vi "Close.vi"(8 "error in (no error)":errorcluster, 11 "MelsecTCP in":refnum<class "Abs Controler.lvclass">) -> (0 "error out":errorcluster, 3 "MelsecTCP out":refnum<class "Abs Controler.lvclass">)   [LabVIEW 2020, in "HslCommunication.lvlib" / "Abs Controler.lvclass"]
uses:
  Abs Controler.lvclass
  E:/Git/Libraries/develop/HslCommunication/_Dependenciecs/HslCommunication.dll
  _Dependenciecs/HslCommunication.dll
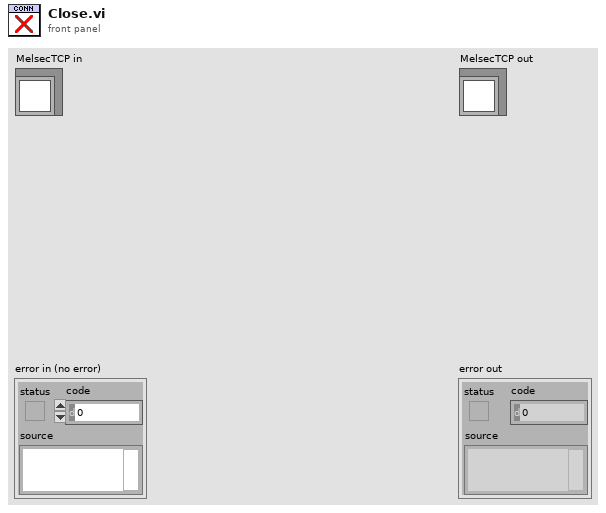
[diagram p1: front panel]
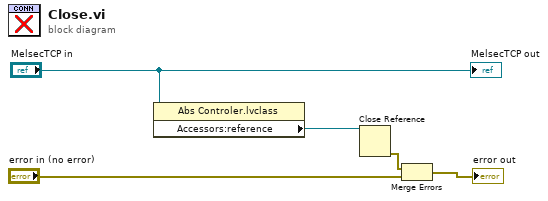
[diagram p0: block diagram]
diagram:
  n1 = property class="Abs Controler.lvclass"(reference="MelsecTCP in") -> ("Accessors:reference"=w3:refnum<k24>)  [unwired: 1 in, 2 out]
  n2 = Close Reference(reference=w3) -> (error out=w1:errorcluster)  [unwired: 1 in]
  n3 = Merge Errors(w1, "error in (no error)") -> (→"error out":errorcluster)
  "MelsecTCP out" <- "MelsecTCP in"
